vi "Choose Camera Implementation.vi"(8 "error in (no error)":errorcluster, 11 "Data Cluster in":T1) -> (0 "error out":errorcluster, 3 "Data Cluster out":T1)   [LabVIEW 2019, in "Camera.lvlib"]
uses:
  Camera.lvlib
  Module Data--cluster.ctl
  Camera-LVClass/Picam_class/Picam.lvclass
  ROI--cluster.ctl
  picam32_LabView_SDK/PICam_lib/types/PicamGatingMode.ctl
  picam32_LabView_SDK/PICam_lib/types/PicamPulse.ctl
  picam32_LabView_SDK/PICam_lib/types/PicamModel.ctl
  <vilib>/Utility/config.llb/Read Key (I32).vi
  <vilib>/Utility/config.llb/NI_LVConfig.lvlib
  picam32_LabView_SDK/PICam_lib/PICam.lvlib
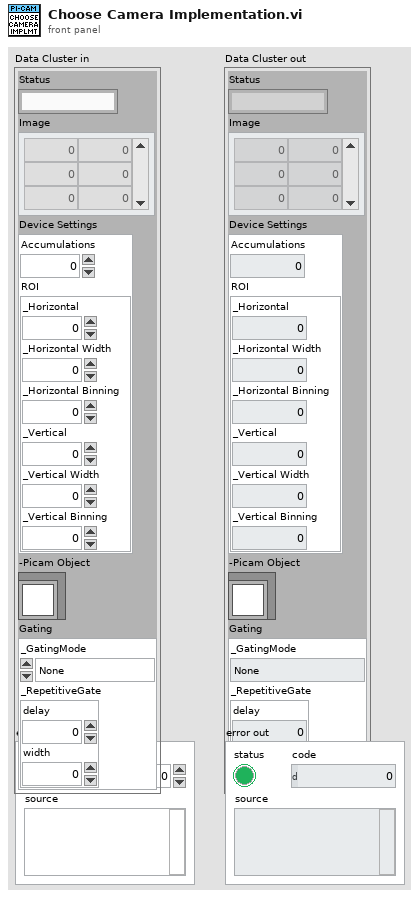
[diagram p1: front panel]
types:
  T1 = typedef "Camera.lvlib/Module Data--cluster.ctl" = cluster{"Status":string, "Image":u16[][], "Device Settings":cluster{"Accumulations":i64, "ROI":T2}, "-Picam Object":refnum<class "Picam.lvclass">, "Gating":cluster{"_GatingMode":T3, "_RepetitiveGate":T4}}
  T2 = typedef "Camera.lvlib/ROI--cluster.ctl" = cluster{"_Horizontal":i32, "_Horizontal Width":i32, "_Horizontal Binning":i32, "_Vertical":i32, "_Vertical Width":i32, "_Vertical Binning":i32}
  T3 = typedef "PICam.lvlib/PicamGatingMode.ctl" = enum16{"None", "Repetitive", "Sequential", "Custom", "Disabled"}
  T4 = typedef "PICam.lvlib/PicamPulse.ctl" = cluster{"delay":dbl, "width":dbl}
  T5 = typedef "NI_LVConfig.lvlib/Config Data RefNum.ctl" = refnum<k1>
  T6 = typedef "PicamModel.ctl" = u32
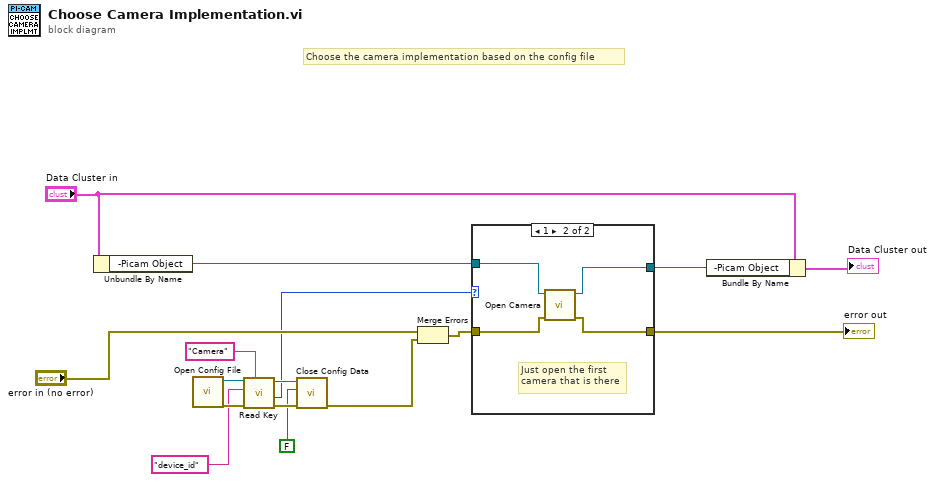
[diagram p0: block diagram]
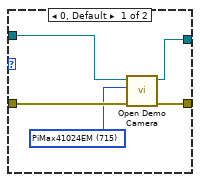
[diagram p2: hidden frame]
diagram:
  # "Choose the camera implementation based on the config file"
  n1 = Unbundle By Name("Data Cluster in") -> ("-Picam Object"=w11:refnum<class "Picam.lvclass">)
  n2 = call "Open Config File.vi"() -> ("error out"=w10:errorcluster, "Refnum out"=w9:T5)  [unwired: 10 in]
  n3 = call-poly <vilib>:"Read Key.vi"("section"="Camera", "error in (no error)"=w10, "key"="device_id", "refnum"=w9) -> ("error out"=w8:errorcluster, "value"=w1:i32, "refnum out"=w7:T5)  [unwired: 4 in, 1 out]
  n4 = call <vilib>:"Close Config Data.vi"("error in (no error)"=w8, "write file if changed (T)"=FALSE, "refnum"=w7) -> ("error out"=w4:errorcluster)  [unwired: 7 in, 1 out]
  n5 = Merge Errors("error in (no error)", w4) -> (w5:errorcluster)
  n6 = case shown="1" w1 {
    tunnel: w5 -> [w21 w23]
    tunnel: [w19 w24] -> w14
    tunnel: [w18 w22] -> w12
    tunnel: w11 -> [w17 w25]
    frame 0, Default {
      w20 = T6 715 items=["---PIXIS 100 SERIES---"=1000, "PixisSeries"=0, "Pixis100BR"=5, "---PI-MAX4 SERIES---"=1001, "Pimax4Series"=700, "PiMax41024EM"=715] ("PicamModel")
      n7 = call-dynamic "Open Demo Camera.vi"("error in (no error)"=w21, "PicamModel"=w20, "Picam in"=w17) -> ("error out"=w18:errorcluster, "Picam out"=w19:refnum<class "Picam.lvclass">)  [unwired: 7 in]
    }
    frame 1 {
      # "Just open the first\ncamera that is there"
      n8 = call-dynamic "Open Camera.vi"("error in (no error)"=w23, "Picam in"=w25) -> ("error out"=w22:errorcluster, "Picam out"=w24:refnum<class "Picam.lvclass">)  [unwired: 7 in, 1 out]
    }
  }
  "error out" <- w12
  n9 = Bundle By Name(cluster="Data Cluster in", "-Picam Object"=w14) -> (→"Data Cluster out":T1)
